vi "MAin_User Login.vi"(7 "error in (no error)":errorcluster caption="에러 입력(에러 없음)", 10 "ID IN":string) -> (0 "error out":errorcluster caption="에러 출력", 1 "권한[0:관리자]":u32, 2 "취소":bool, 3 "ID OUT":string)   [LabVIEW 2019]
uses:
  cmd_logInfor.ctl
  <vilib>/Utility/config.llb/Read Key (String).vi
  <vilib>/Utility/config.llb/Read Key (U32).vi
  <vilib>/Utility/config.llb/NI_LVConfig.lvlib
panel:
  in  "사용자 등록":bool
  in  "exit":bool
  in  "login":bool
  in  "pw":string caption="PW"
  in  "id":string caption="ID"
  # "User Log-In"
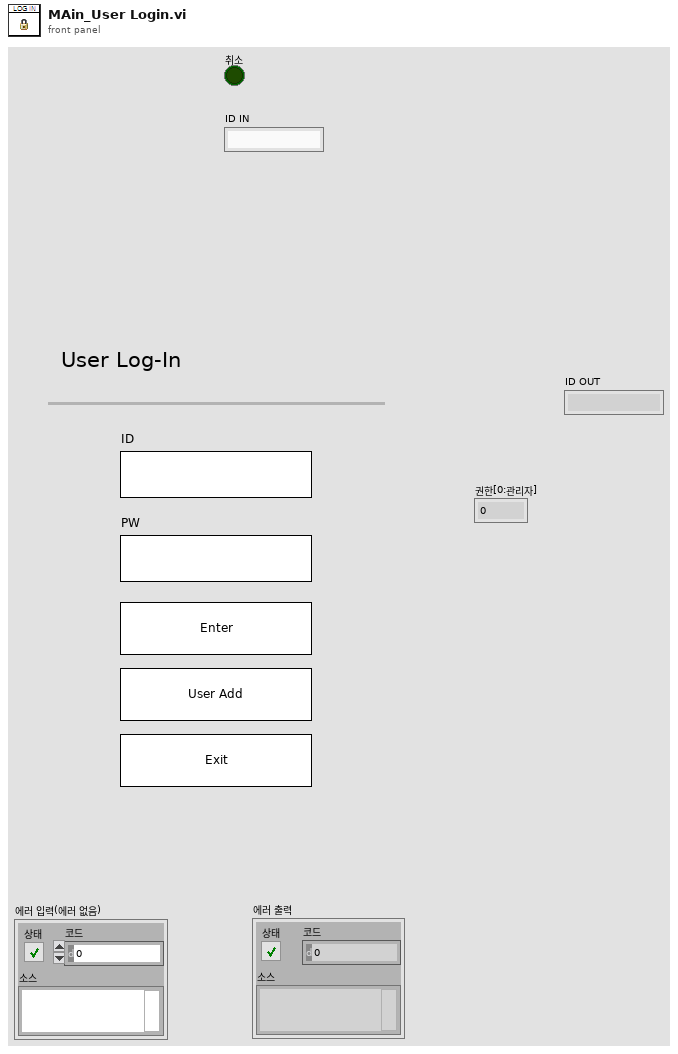
[diagram p1: front panel]
types:
  T1 = typedef "cmd_logInfor.ctl" = enum16{"ADMIN", "OPER", "DEFAULT"}
  T2 = typedef "NI_LVConfig.lvlib/Config Data RefNum.ctl" = refnum<k1>
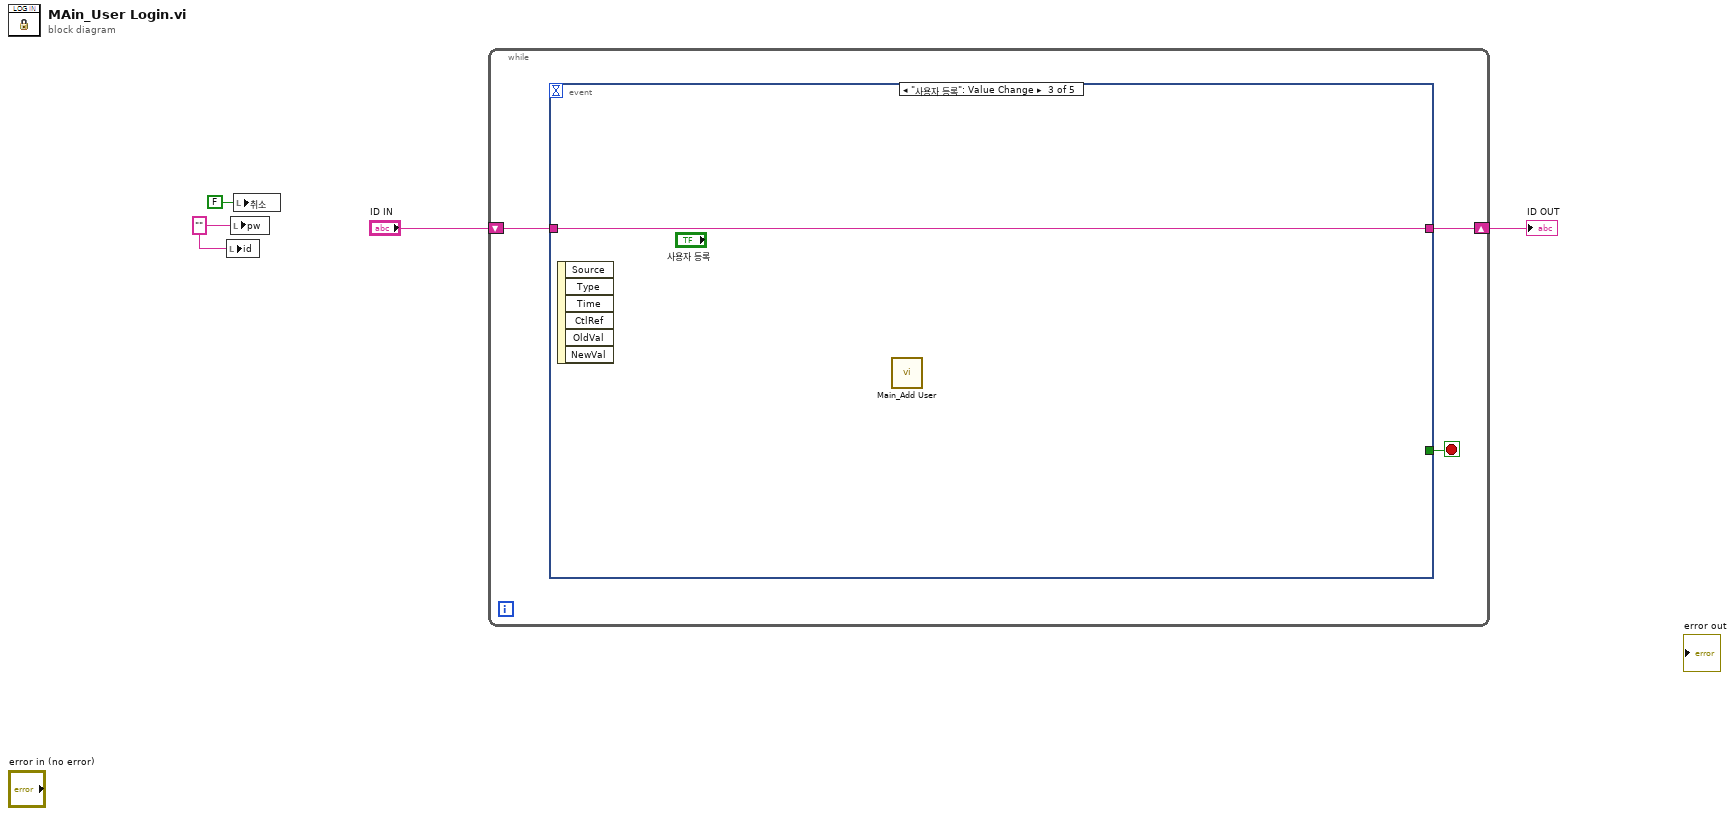
[diagram p0: block diagram]
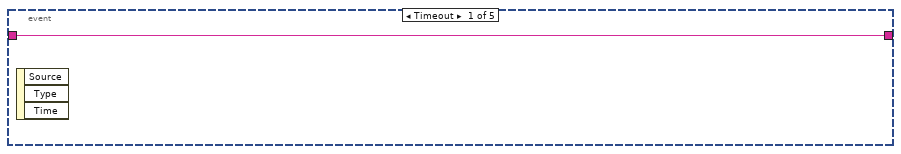
[diagram p2: hidden frame]
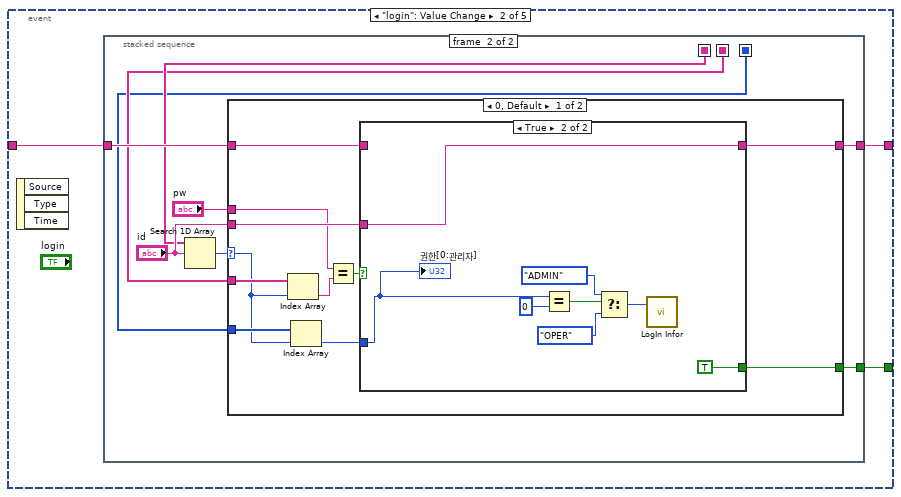
[diagram p3: hidden frame]
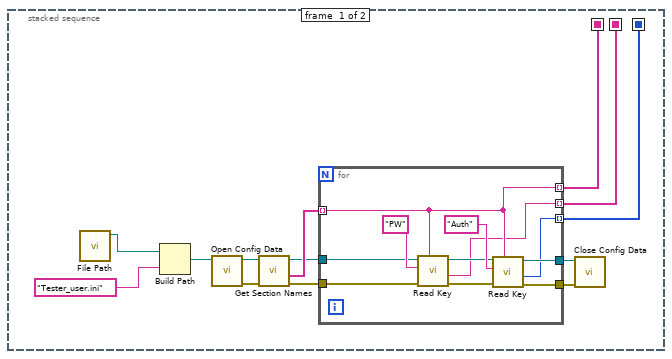
[diagram p4: hidden frame]
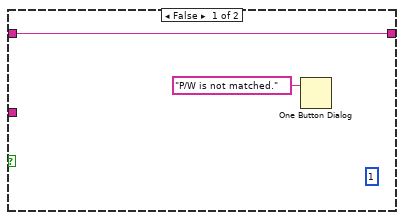
[diagram p5: hidden frame]
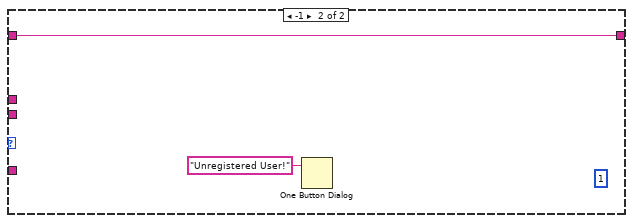
[diagram p6: hidden frame]
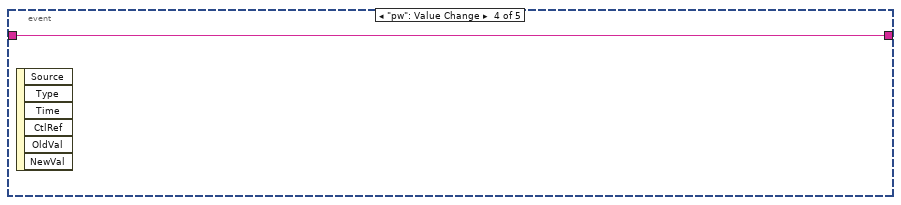
[diagram p7: hidden frame]
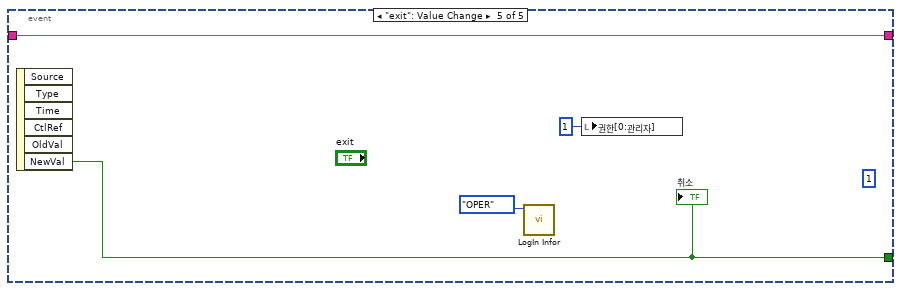
[diagram p8: hidden frame]
diagram:
  w4 = "" ("문자열 2")
  n1 = local write "id"(w4) -> ()
  n2 = local write "pw"(w4) -> ()
  n3 = local write "취소"(FALSE ("새 값")) -> ()
  n4 = while {
    shift-right: [w6] -> w1
    shift-left: "ID IN" -> [w5]
    stop <- w7 stop-if-true
    n5 = event shown="[2] \"사용자 등록\": Value Change" {
      selector: _ -> [_ _ _ _ _]
      dyn-events: _ -> [_ _ _ _ _]
      timeout: _ -> [_ _ _ _ _]
      tunnel: [_ w11 _ _ w73] -> w7
      tunnel: w5 -> [w8 w9 w68 w69 w72]
      tunnel: [w8 w10 w68 w69 w72] -> w6
      event Timeout {
        n6 = event-data() -> ()  [unwired: 1 in, 3 out]
      }
      event "login": Value Change {
        n7 = event-data() -> ()  [unwired: 1 in, 3 out]
        n8 = stacked-sequence {
          seq-local: [w15 _] -> [_ w38]
          seq-local: [w14 _] -> [_ w37]
          seq-local: [w13 _] -> [_ w36]
          tunnel: [_ w43] -> w11
          tunnel: [_ w40] -> w10
          tunnel: w9 -> [_ w39]
          frame #0 {
            n9 = call "File Path.vi"() -> ("condition"=w12:path)  [unwired: 7 in, 4 out]
            n10 = Build Path(base path=w12, name or relative path="Tester_user.ini" ("이름 또는 상대 경로")) -> (appended path=w24:path)
            n11 = call <vilib>:"Open Config Data.vi"("configuration file path"=w24) -> ("error out"=w21:errorcluster, "refnum"=w19:T2)  [unwired: 8 in, 1 out]
            n12 = call <vilib>:"Get Section Names.vi"("error in (no error)"=w21, "refnum"=w19) -> ("error out"=w22:errorcluster, "section names"=w23:string[], "refnum out"=w20:T2)  [unwired: 7 in]
            n13 = for {
              tunnel: [w35] -> w17
              tunnel: [w34] -> w18
              tunnel: w20 -> [w29]
              tunnel: w22 -> [w28]
              tunnel: w23 -> [w27] mode=indexing
              tunnel: [w27] -> w15 mode=indexing
              tunnel: [w26] -> w14 mode=indexing
              tunnel: [w25] -> w13 mode=indexing
              n14 = call-poly <vilib>:"Read Key.vi"("section"=w27, "error in (no error)"=w28, "key"="PW", "refnum"=w29) -> ("error out"=w31:errorcluster, "value"=w26:string, "refnum out"=w30:T2)  [unwired: 4 in, 1 out]
              n15 = call-poly <vilib>:"Read Key.vi"("section"=w27, "error in (no error)"=w31, "key"="Auth" ("default value"), "refnum"=w30) -> ("error out"=w35:errorcluster, "value"=w25:u32, "refnum out"=w34:T2)  [unwired: 4 in, 1 out]
            }
            n16 = call <vilib>:"Close Config Data.vi"("error in (no error)"=w17, "refnum"=w18) -> ()  [unwired: 8 in, 2 out]
          }
          frame #1 {
            n17 = Search 1D Array(1D array=w38, element="id") -> (index of element=w44:i32)  [unwired: 1 in]
            n18 = case shown="0, Default" w44 {
              selector: w44 -> [w49 _]
              tunnel: w37 -> [w55 _]
              tunnel: [w52 _] -> w43
              tunnel: "id" -> [w51 _]
              tunnel: w36 -> [w50 _]
              tunnel: "pw" -> [w47 _]
              tunnel: [w46 w66] -> w40
              tunnel: w39 -> [w45 w66]
              frame 0, Default {
                n19 = Index Array(array=w55, index=w49) -> (element=w54:string)
                n20 = Index Array(array=w50, index=w49) -> (element=w48:u32)
                n21 = Equal?(x=w47, y=w54) -> (x = y?=w53:bool)
                n22 = case shown="True" w53 {
                  tunnel: [_ TRUE] -> w52
                  tunnel: w51 -> [_ w64]
                  tunnel: w48 -> [_ w58]
                  tunnel: [w56 w64] -> w46
                  tunnel: w45 -> [w56 _]
                  frame False {
                    (unwired) u32 1 ("value")
                    n23 = One Button Dialog(message="P/W is not matched." ("메시지")) -> ()  [unwired: 1 in, 1 out]
                  }
                  frame True {
                    n24 = Equal?(x=w58, y=u32 0) -> (x = y?=w60:bool)
                    n25 = Select(t=cmd_logInfor."ADMIN" ("USER IN"), s=w60, f=cmd_logInfor."OPER" ("USER IN")) -> (s? t:f=w63:T1)
                    n26 = call "LogIn Infor.vi"("USER IN"=w63) -> ()  [unwired: 8 in, 3 out]
                    "권한[0:관리자]" <- w58
                  }
                }
              }
              frame -1 {
                (unwired) u32 1 ("value")
                n27 = One Button Dialog(message="Unregistered User!" ("메시지")) -> ()  [unwired: 1 in, 1 out]
              }
            }
          }
        }
      }
      event "사용자 등록": Value Change {
        n28 = event-data() -> ()  [unwired: 1 in, 6 out]
        n29 = call "Main_Add User.vi"() -> ()  [unwired: 11 in, 1 out]
      }
      event "pw": Value Change {
        n30 = event-data() -> ()  [unwired: 1 in, 6 out]
      }
      event "exit": Value Change {
        (unwired) u32 1 ("value")
        n31 = event-data() -> ("NewVal"=w73:bool)  [unwired: 1 in, 5 out]
        "취소" <- w73
        n32 = call "LogIn Infor.vi"("USER IN"=cmd_logInfor."OPER") -> ()  [unwired: 8 in, 3 out]
        n33 = local write "권한[0:관리자]"(u32 1 ("권한[0:관리자]")) -> ()
      }
    }
  }
  "ID OUT" <- w1
